vi "S8300E_shutdown_UUT_WIH.vi"() -> ()   [LabVIEW 2011]
panel:
  out "SHUTDOWN_TIMEOUT":string
  out "log1":string
  out "Debug View":string
  out "VISA resource name out":refnum<visa-resource-name>
  out "進行狀況":string
  out "BEGIN TIME":u32
  # "2015-5-28"
  # "Error Code:MB-NG"
  # "S8300E ShutDown  UUT"
  # "COM9 115200"
  # "Delay 0.5 sec after get power down from Console"
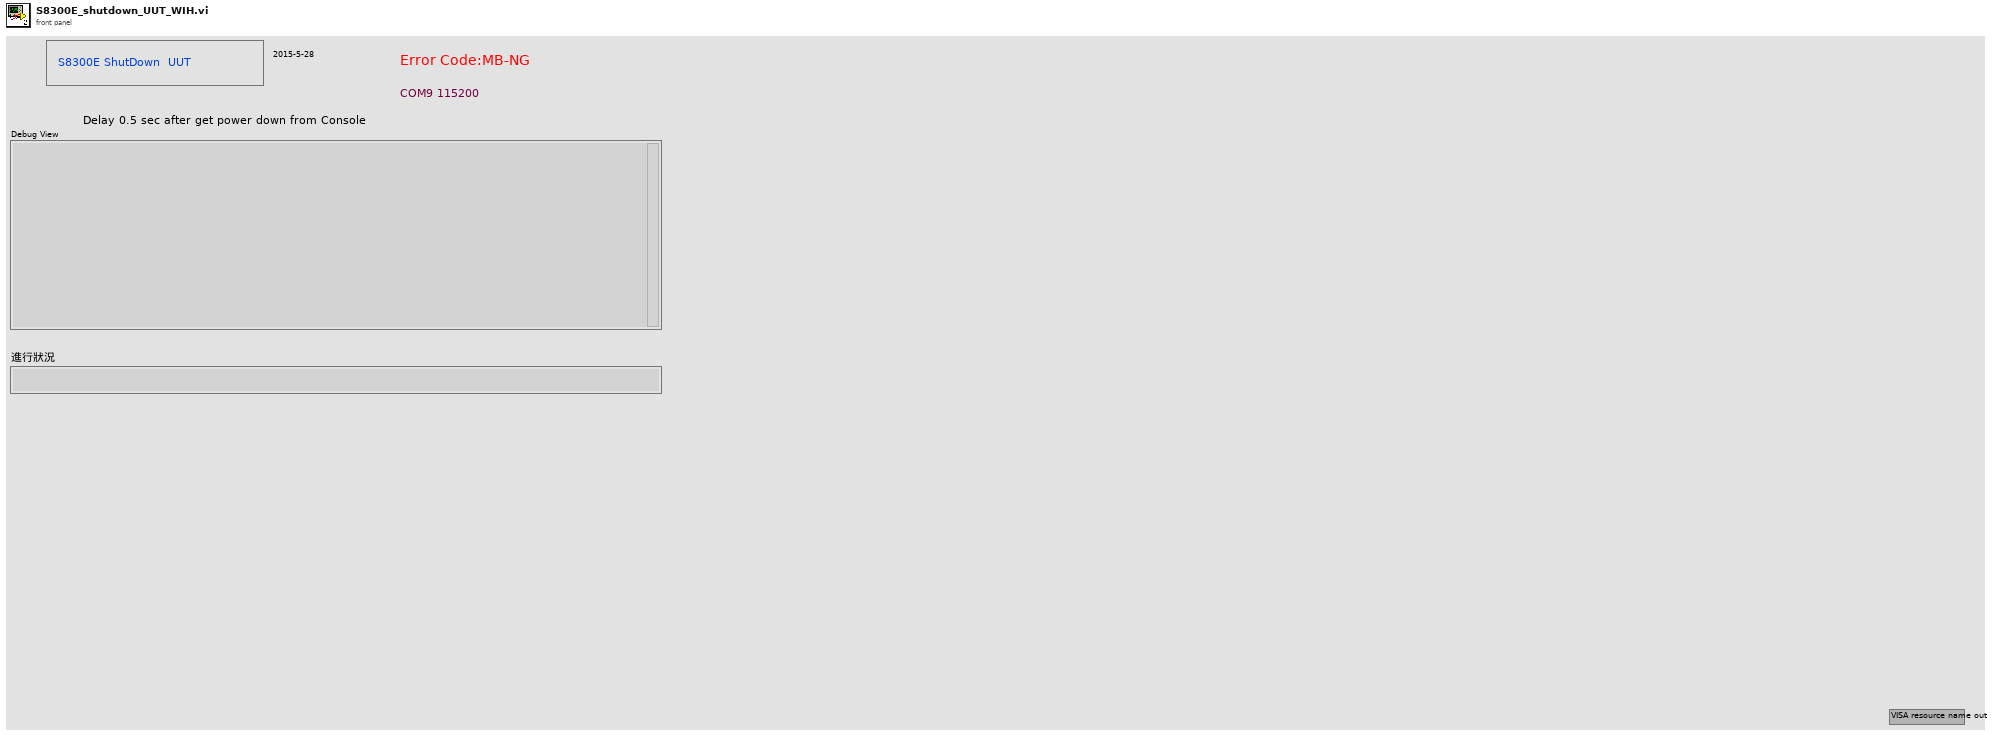
[diagram p1: front panel]
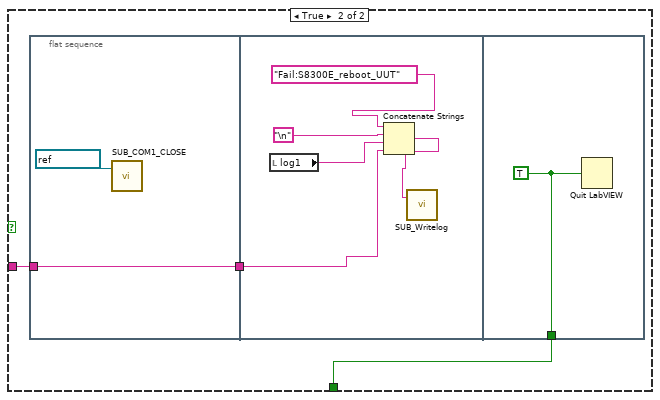
[diagram p6: hidden frame]
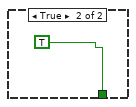
[diagram p7: hidden frame]
diagram:
  n1 = flat-sequence {
    tunnel: [w21] -> w3
    tunnel: [w24] -> w2
    tunnel: w3 -> [w29]
    tunnel: w2 -> [w28]
    tunnel: [w26] -> w1
    tunnel: w1 -> [w48]
    frame #0 {
      n2 = Tick Count (ms)() -> (millisecond timer value=→"BEGIN TIME":u32)
    }
    frame #1 {
      n3 = call "SUB_COM1_CLOSE.vi"("VISA resource name"=refnum<visa-resource-name> "COM9") -> ()  [unwired: 3 in]
      n4 = property on="進行狀況" class="Str"("Blinking"=TRUE) -> ()  [unwired: 2 in, 2 out]
      "進行狀況" <- "進入測試準備中...." ("進行狀況")
      "Debug View" <- ""
    }
    frame #2 {
      n5 = call "SUB_SearchFile_inFolder.vi"("Search Filename in Folder"="S8300E_sfcs_misc.txt") -> ("File Existing True/Flase"=w9:bool)  [unwired: 1 in]
      n6 = case shown="False" w9 {
        frame False {
          n7 = flat-sequence {
            frame #0 {
              n8 = call "Display Message to User2"() -> ()  [unwired: 10 in, 2 out]
            }
            frame #1 {
              n9 = call "SUB_Writelog.vi"("Pass/Fail"="Fail:S8300E_shutdown_UUT_WIH") -> ()  [unwired: 2 in]
            }
            frame #2 {
              n10 = Quit LabVIEW(quit? (T)=TRUE) -> ()
            }
          }
        }
        frame True {
        }
      }
    }
    frame #3 {
      n11 = call "SUB_Read_specifFile.vi"("name or relative path"="S8300E_sfcs_misc.txt" ("Search Filename in Folder")) -> ("text"=w16:string)  [unwired: 1 in, 1 out]
      n12 = call "SUB_FindSpecificString.vi"("Find this String"="SHUTDOWN_TIMEOUT__SEC=", "String data"=w16) -> ("before \"; \" string"=→"SHUTDOWN_TIMEOUT":string, "Found"=w14:bool)  [unwired: 2 in]
      n13 = case shown="False" w14 {
        frame False {
          n14 = flat-sequence {
            frame #0 {
              n15 = call "Display Message to User3"() -> ()  [unwired: 10 in, 2 out]
            }
            frame #1 {
              n16 = call "SUB_Writelog.vi"("Pass/Fail"="Fail:S8300E_shutdown_UUT_WIH") -> ()  [unwired: 2 in]
            }
            frame #2 {
              n17 = Quit LabVIEW(quit? (T)=TRUE) -> ()
            }
          }
        }
        frame True {
        }
      }
    }
    frame #4 {
      n18 = call "SUB_COM9_INIT.vi"("baud rate"=u32 115200) -> ("VISA resource name out"=w21:refnum<visa-resource-name>)  [unwired: 1 in, 1 out]
      "VISA resource name out" <- w21
      n19 = call "SUB_COM1Wrt.vi"("VISA resource name"=w21, "write buffer"="\r") -> ("duplicate VISA resource name"=w20:refnum<visa-resource-name>)  [unwired: 1 in, 1 out]
      n20 = Tick Count (ms)() -> (millisecond timer value=w24:u32)
      n21 = call "SUB_ContinueCom1Read.vi"("Numeric"=9600, "duplicate VISA resource name 2"=w20) -> ()  [unwired: 1 in, 3 out]
    }
    frame #5 {
      n22 = while {
        tunnel: w29 -> [w44]
        tunnel: w28 -> [w42]
        shift-right: [w31] -> _
        shift-left: "" -> [w36]
        tunnel: [w32] -> w26
        stop <- w35 stop-if-true
        n23 = Tick Count (ms)() -> (millisecond timer value=w43:u32)
        n24 = call "SUB_COM1Wrt.vi"("VISA resource name"=w44, "write buffer"="\r") -> ("duplicate VISA resource name"=w45:refnum<visa-resource-name>)  [unwired: 1 in, 1 out]
        n25 = Subtract(x=w43, y=w42) -> (x-y=w41:u32)
        n26 = Divide(x=w41, y=u32 1000) -> (x/y=w39:dbl)
        n27 = Wait (ms)(milliseconds to wait=u32 50) -> ()  [unwired: 1 out]
        n28 = Greater Or Equal?(x=w39, y=5.0) -> (x >= y?=w34:bool)
        n29 = call "SUB_ContinueCom1Read.vi"("Numeric"=50, "duplicate VISA resource name 2"=w45) -> ("String"=w37:string)  [unwired: 1 in, 2 out]
        n30 = Concatenate Strings(w36, w37) -> (w31:string)
        n31 = call "SUB_FindSpecificString.vi"("Find this String"="root@", "String data"=w31) -> ("Found"=w32:bool)  [unwired: 2 in, 1 out]
        n32 = local write "Debug View"(w31) -> ()
        n33 = Or(x=w32, y=w34) -> (x .or. y?=w35:bool)
      }
    }
    frame #6 {
      n34 = case shown="False" w48 {
        frame False {
          w51 = "root@" ("Find this String")
          n35 = Tick Count (ms)() -> (millisecond timer value=w53:u32)
          n36 = local read "VISA resource name out"() -> (w55:refnum<visa-resource-name>)
          n37 = call "SUB_COM1Wrt.vi"("VISA resource name"=w55, "write buffer"="\r") -> ("duplicate VISA resource name"=w54:refnum<visa-resource-name>)  [unwired: 1 in, 1 out]
          n38 = call "SUB_READ_COM1_FindString_timeout.vi"("Find this String"=w51, "Timeout Seccond"=6.0, "Begin time"=w53, "duplicate VISA resource name 2"=w54) -> ("Output String"=w50:string)  [unwired: 1 in, 2 out]
          n39 = call "SUB_FindSpecificString.vi"("Find this String"=w51, "String data"=w50) -> ("Found"=w49:bool)  [unwired: 2 in, 1 out]
          n40 = case shown="False" w49 {
            tunnel: w50 -> [w59 _]
            frame False {
              n41 = flat-sequence {
                tunnel: w59 -> [w61]
                tunnel: [w60] -> w57
                tunnel: [w64] -> w58
                tunnel: w57 -> [w64]
                tunnel: w58 -> [w67]
                frame #0 {
                  n42 = Concatenate Strings("系統需在Test Mode 下,有root 權限!" ("string"), "\n", w61) -> (w60:string)
                  n43 = call "Display Message to User"("Message"=w60) -> ()  [unwired: 9 in, 2 out]
                }
                frame #1 {
                  n44 = call "SUB_COM1_CLOSE.vi"("VISA resource name"=refnum<visa-resource-name> "COM9") -> ()  [unwired: 3 in]
                }
                frame #2 {
                  n45 = Concatenate Strings("Fail:S8300E_shutdown_UUT" ("Pass/Fail"), "\n", w67) -> (w66:string)
                  n46 = call "SUB_Writelog.vi"("Pass/Fail"=w66) -> ()  [unwired: 2 in]
                }
                frame #3 {
                  n47 = Quit LabVIEW(quit? (T)=TRUE) -> ()
                }
              }
            }
            frame True {
            }
          }
        }
        frame True {
        }
      }
    }
    frame #7 {
      w74 = "\r"
      n48 = local read "VISA resource name out"() -> (w75:refnum<visa-resource-name>)
      n49 = call "SUB_ContinueCom1Read.vi"("Numeric"=4800, "duplicate VISA resource name 2"=w75) -> ("duplicate VISA resource name"=w71:refnum<visa-resource-name>)  [unwired: 1 in, 2 out]
      n50 = Concatenate Strings("shutdown -h now" ("string"), w74, w74) -> (w73:string)
      n51 = call "SUB_COM1Wrt.vi"("VISA resource name"=w71, "write buffer"=w73) -> ()  [unwired: 1 in, 2 out]
    }
    frame #8 {
      n52 = Wait (ms)(milliseconds to wait=u32 2000) -> ()  [unwired: 1 out]
    }
    frame #9 {
      n53 = while {
        shift-right: [w84] -> _
        shift-left: "" -> [w83]
        stop <- w88 stop-if-true
        n54 = local read "SHUTDOWN_TIMEOUT"() -> (w80:string)
        n55 = local read "VISA resource name out"() -> (w81:refnum<visa-resource-name>)
        n56 = Tick Count (ms)() -> (millisecond timer value=w85:u32)
        n57 = Fract/Exp String To Number(string=w80) -> (number=w79:dbl)  [unwired: 3 in, 1 out]
        n58 = call "SUB_READ_COM1_FindString_timeout.vi"("Find this String"="reboot: Power down", "Timeout Seccond"=w79, "Begin time"=w85, "duplicate VISA resource name 2"=w81) -> ("Output String"=w82:string, "Found String"=w86:bool)  [unwired: 1 in, 1 out]
        n59 = local write "Debug View"(w82) -> ()
        n60 = case shown="False" w86 {
          tunnel: w82 -> [w94 _]
          tunnel: [w90 TRUE] -> w88
          tunnel: w82 -> [w89 _]
          frame False {
            n61 = call "SUB_YESNO.vi"("Debug View"=w94, "Status"="UART沒反應!") -> ("yes/no"=w93:enum32{"No Selection", "Yes", "No", "None"})  [unwired: 1 in]
            n62 = Equal?(x=w93, y=enum32{"No Selection", "Yes", "No", "None"}."No") -> (x = y?=w91:bool)
            n63 = case shown="False" w91 {
              tunnel: [_ w102] -> w90
              tunnel: w89 -> [_ w100]
              frame False {
                w99 = "\r"
                n64 = local read "VISA resource name out"() -> (w96:refnum<visa-resource-name>)
                n65 = Concatenate Strings("shutdown -h now" ("string"), w99, w99) -> (w98:string)
                n66 = call "SUB_COM1Wrt.vi"("VISA resource name"=w96, "write buffer"=w98) -> ()  [unwired: 1 in, 2 out]
              }
              frame True {
                n67 = flat-sequence {
                  tunnel: [w103] -> w101
                  tunnel: w100 -> [w103]
                  tunnel: w101 -> [w105]
                  tunnel: [w110] -> w102
                  frame #0 {
                    n68 = call "SUB_COM1_CLOSE.vi"("VISA resource name"=refnum<visa-resource-name> "COM9") -> ()  [unwired: 3 in]
                  }
                  frame #1 {
                    n69 = local read "log1"() -> (w106:string)
                    n70 = Concatenate Strings("Fail:S8300E_reboot_UUT" ("Pass/Fail"), "\n", w106, w105) -> (w107:string)
                    n71 = call "SUB_Writelog.vi"("Pass/Fail"=w107) -> ()  [unwired: 2 in]
                  }
                  frame #2 {
                    w110 = TRUE ("quit? (T)")
                    n72 = Quit LabVIEW(quit? (T)=w110) -> ()
                  }
                }
              }
            }
          }
          frame True {
          }
        }
        n73 = Concatenate Strings(w83, w82) -> (w84:string)
        "log1" <- w84
      }
    }
    frame #10 {
      n74 = Wait (ms)(milliseconds to wait=u32 500) -> ()  [unwired: 1 out]
    }
    frame #11 {
      w115 = "\r"
      n75 = Tick Count (ms)() -> (millisecond timer value=w119:u32)
      n76 = local read "BEGIN TIME"() -> (w120:u32)
      n77 = local read "Debug View"() -> (w116:string)
      n78 = call "SUB_COM1_CLOSE.vi"("VISA resource name"=refnum<visa-resource-name> "COM9") -> ()  [unwired: 3 in]
      n79 = call "SUB_CAL_TESTTIME.vi"("Test Item name"="S8300E_shutdown_UUT", "Stop tick time"=w119, "Start tick time"=w120) -> ("Test Time output"=w114:string)  [unwired: 2 in]
      n80 = Concatenate Strings("Pass:S8300E_shutdown_UUT" ("string"), w115, w116, w115, w114) -> (w117:string)
      n81 = call "SUB_Writelog.vi"("Pass/Fail"=w117) -> ()  [unwired: 2 in]
    }
    frame #12 {
      n82 = Request Deallocation(TRUE ("flag")) -> ()
    }
    frame #13 {
      n83 = Quit LabVIEW(quit? (T)=TRUE) -> ()
    }
  }
